vi "Generate Waveform (Multi-Array).vi"(0 "number of samples":u32=300000 caption="Number of Samples", 5 "sample rate":dbl=10000000.0 caption="Sample Rate" format="%#.3pS/s", 7 "tone frequency":dbl=130000.0 caption="Tone Frequency" format="%#.3pHz", 9 "amplitude":dbl=1.0 caption="Amplitude" format="%#.6g") -> (4 "I":i16[](array[numeric]), 6 "Q":i16[](array[numeric]), 8 "Waveform":waveform(dbl)[](graph))   [LabVIEW 2013]
doc: "Creates a waveform to send to a device for generation.\n\n<B>Input Parameters</B>\n\n<B>number of samples</B> in the generated waveform.\n\n<B>sample rate</B> is the rate, in samples per second, that will be used to create the waveform.\n\n<B>tone frequency</B> is the frequency of the tone, in hertz, to generate.\n\n<B>amplitude</B> is used to set the amplitude of the tone. DSP overflow will occur if the 'amplitude' is too high.\n\n<B>Output Parameters</B>\n\n<B>I</B> is the real (I) portion of the generated waveform.\n\n<B>Q</B> is the imaginary (Q) portion of the generated waveform.\n\n<B>Waveform</B> is the generated waveform."
uses:
  <vilib>/measure/NI_MABase.lvlib
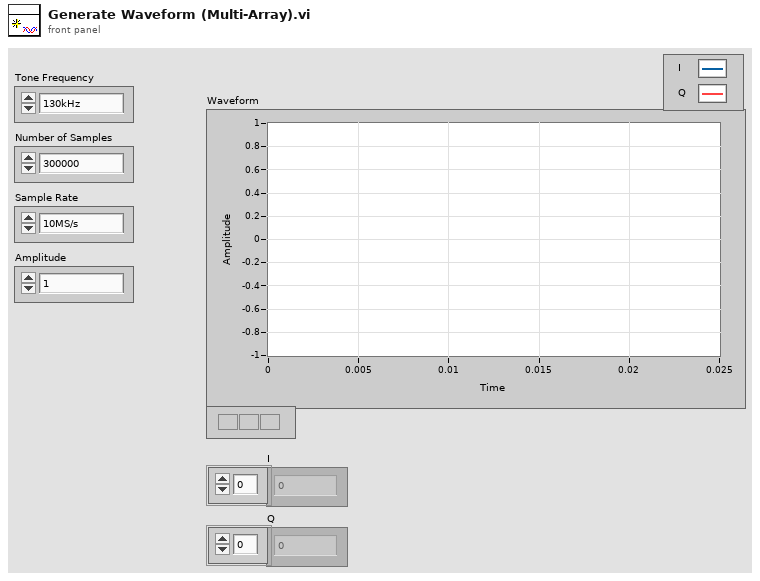
[diagram p1: front panel]
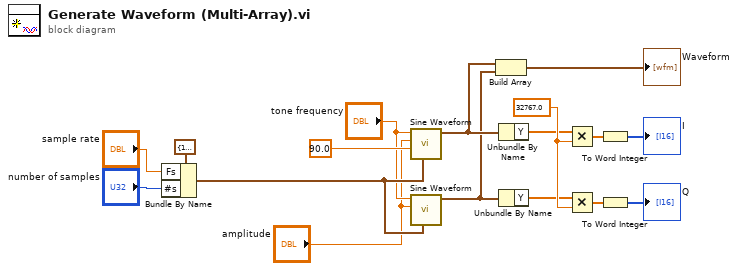
[diagram p0: block diagram]
diagram:
  w13 = 32767.0
  n1 = Bundle By Name(cluster=cluster{"Fs":dbl, "#s":dbl} {"Fs"=1000.0, "#s"=1000.0} ("sampling info"), "Fs"="sample rate", "#s"="number of samples") -> (w9:cluster{"Fs":dbl, "#s":dbl})
  n2 = call <vilib>:"Sine Waveform.vi"("sampling info"=w9, "phase"=90.0, "amplitude"="amplitude", "frequency"="tone frequency") -> ("signal out"=w7:waveform(dbl))  [unwired: 6 in, 1 out]
  n3 = call <vilib>:"Sine Waveform.vi"("sampling info"=w9, "amplitude"="amplitude", "frequency"="tone frequency") -> ("signal out"=w6:waveform(dbl))  [unwired: 7 in, 1 out]
  n4 = Build Array(w7, w6) -> (→"Waveform":waveform(dbl)[])
  n5 = Unbundle By Name(w7) -> ("Y"=w11:dbl[])
  n6 = Unbundle By Name(w6) -> ("Y"=w12:dbl[])
  n7 = Multiply(x=w11, y=w13) -> (x*y=w14:dbl[])
  n8 = Multiply(x=w12, y=w13) -> (x*y=w15:dbl[])
  n9 = To Word Integer(number=w14) -> (16bit integer=→"I":i16[])
  n10 = To Word Integer(number=w15) -> (16bit integer=→"Q":i16[])
